vi "GET.vi"(6 "timeout":i32=10000, 7 "output file":path, 8 "error in":errorcluster, 10 "url":string, 11 "http-method in":refnum<class "net-http-client.lvclass">) -> (0 "error out":errorcluster, 2 "response":refnum<class "response.lvclass">, 3 "http-method out":refnum<class "net-http-client.lvclass">)   [LabVIEW 2020, in "net-http-client.lvclass"]
uses:
  net-http-client.lvclass
  classes/response/response.lvclass
  <vilib>/Viviota/Viviota HTTP Client NET/Types/method_enum.ctl
  net-http-client.lvclass/net-http-client.ctl
  <vilib>/Viviota/Viviota HTTP Client NET/LabVIEWHTTPClient_NET/HttpClient_NET.lvclass
  <vilib>/Viviota/Viviota HTTP Client NET/HttpClient_NET.lvlib
  net-response/net-response.lvclass
panel:
  out "Timeout":bool
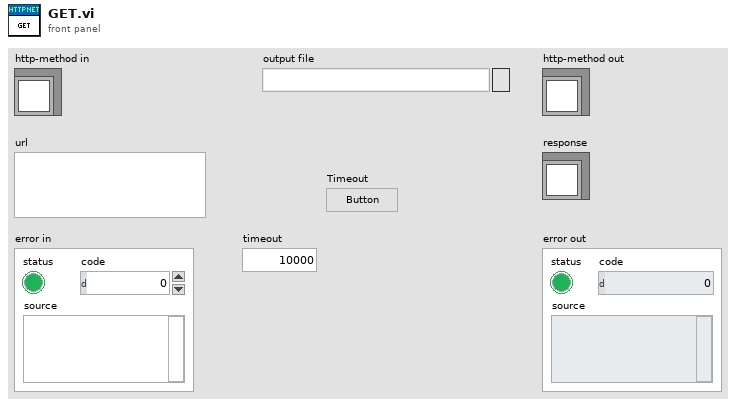
[diagram p1: front panel]
types:
  T1 = typedef "HttpClient_NET.lvlib/method_enum.ctl" = enum16{"GET", "PUT", "POST", "DELETE", "HEAD", "TRACE", "SEND"}
  T2 = typedef "HttpClient_NET.lvlib/ResponseHeaders_Cluster.ctl" = cluster{"ResponseHeader":refnum<class "HttpHeaders_Response.lvclass">, "ContentHeaders":refnum<class "HttpHeaders_Content.lvclass">}
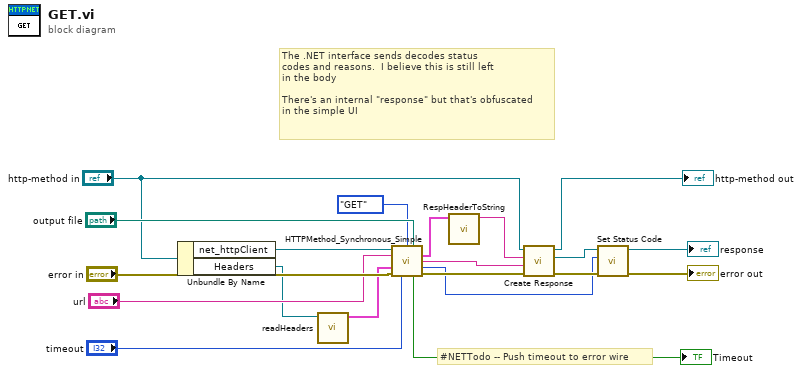
[diagram p0: block diagram]
diagram:
  # "#NETTodo -- Push timeout to error wire"
  # "The .NET interface sends decodes status\ncodes and reasons.  I believe this is still left\nin the body\n\nThere's an internal \"response\" but that's obfuscated\nin the simple UI"
  n1 = Unbundle By Name("http-method in") -> ("net_httpClient"=w15:refnum<class "HttpClient_NET.lvclass">, "Headers"=w2:refnum<data-value>)
  n2 = call "readHeaders.vi"("HeaderRef In"=w2) -> ("Headers"=w1:cluster{"key":string, "value":string}[])  [unwired: 10 in]
  n3 = call <vilib>:"HTTPMethod_Synchronous_Simple.vi"("LabVIEWHTTPClient_NET in"=w15, "Method"=method_enum."GET", "output file"="output file", "URL"="url", "request headers"=w1, "error in (no error)"="error in", "Timeout_ms (10000)"="timeout") -> ("Headers"=w9:T2, "Response"=w10:string, "StatusCode"=w3:i32, "Timeout"=→"Timeout":bool, "error out"=w13:errorcluster)  [unwired: 2 in, 2 out]
  n4 = call "RespHeaderToString.vi"("Headers"=w9) -> ("HeaderString"=w8:string)  [unwired: 10 in]
  n5 = call-dynamic "Create Response.vi"("error in (no error)"=w13, "body"=w10, "headers"=w8, "http-client"="http-method in") -> ("error out"=w5:errorcluster, "response"=w7:refnum<class "response.lvclass">, "http-client out"=→"http-method out":refnum<class "net-http-client.lvclass">)  [unwired: 5 in]
  n6 = call "Set Status Code.vi"("error in (no error)"=w5, "StatusCode"=w3, "net-response in"=w7) -> ("error out"=→"error out":errorcluster, "net-response out"=→"response":refnum<class "response.lvclass">)  [unwired: 7 in]
